vi "Do 6-Contact Sample Hall Calculations.vi"(8 "error in (no error)":errorcluster) -> (0 "error out":errorcluster)   [LabVIEW 2016, in "Hall Effect Library.lvlib"]
uses:
  Hall Effect Library.lvlib
  Global Variables/Hall Effect Data.vi
  Global Variables/Test Settings.vi
panel:
  out "uH":dbl
  out "Ravg":dbl
  out "Rh2":dbl
  out "Rh1":dbl
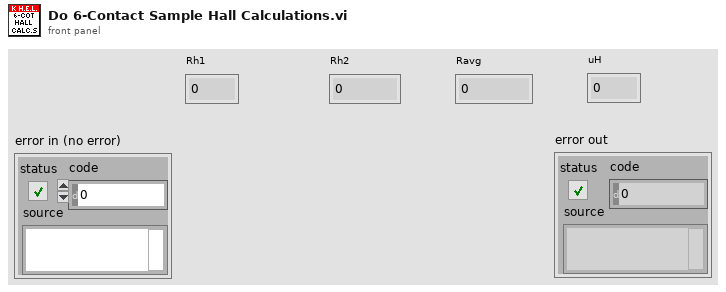
[diagram p1: front panel]
types:
  T1 = cluster{"RAvg":dbl, "RH1":dbl, "RH2":dbl, "uH":dbl}
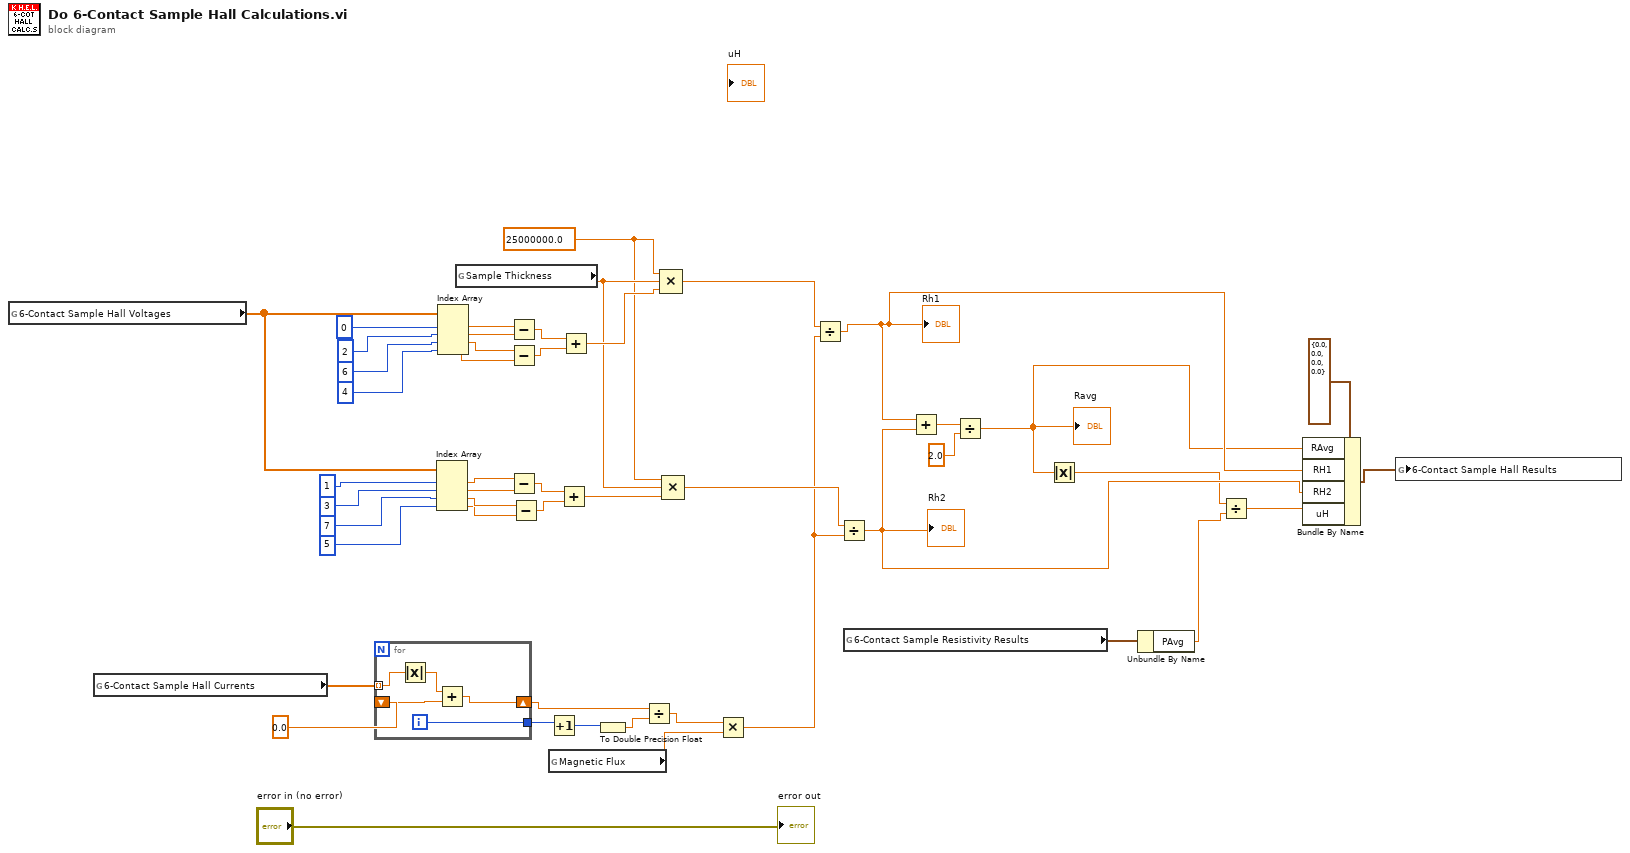
[diagram p0: block diagram]
diagram:
  w17 = 25000000.0
  n1 = global read "Hall Effect Data.vi" "6-Contact Sample Hall Voltages"() -> (w30:dbl[])
  n2 = global read "Hall Effect Data.vi" "6-Contact Sample Hall Currents"() -> (w46:dbl[])
  n3 = for {
    shift-right: [w52] -> w42
    shift-left: 0.0 -> [w53]
    tunnel: w46 -> [w50] mode=indexing
    tunnel: [w51] -> w45
    i -> [w51]
    n4 = Absolute Value(x=w50) -> (abs(x)=w49:dbl)
    n5 = Add(x=w49, y=w53) -> (x+y=w52:dbl)
  }
  n6 = Index Array(array=w30, index #1=1, index #2=3, index #3=7, index #4=5) -> (element #1=w25:dbl, element #2=w24:dbl, element #3=w23:dbl, element #4=w22:dbl)
  n7 = Index Array(array=w30, index #1=0, index #2=2, index #3=6, index #4=4) -> (element #1=w37:dbl, element #2=w36:dbl, element #3=w35:dbl, element #4=w34:dbl)
  n8 = global read "Test Settings.vi" "Sample Thickness"() -> (w18:dbl)
  n9 = Subtract(x=w37, y=w36) -> (x-y=w33:dbl)
  n10 = Subtract(x=w35, y=w34) -> (x-y=w32:dbl)
  n11 = Subtract(x=w25, y=w24) -> (x-y=w21:dbl)
  n12 = Subtract(x=w23, y=w22) -> (x-y=w20:dbl)
  n13 = Increment(x=w45) -> (x+1=w44:i32)
  n14 = global read "Test Settings.vi" "Magnetic Flux"() -> (w15:dbl)
  n15 = Add(x=w21, y=w20) -> (x+y=w19:dbl)
  n16 = Add(x=w33, y=w32) -> (x+y=w31:dbl)
  n17 = To Double Precision Float(number=w44) -> (double precision float=w43:dbl)
  n18 = Divide(x=w42, y=w43) -> (x/y=w16:dbl)
  n19 = Compound Arithmetic op=MULTIPLY(w17, w18, w31) -> (w14:dbl)
  n20 = Compound Arithmetic op=MULTIPLY(w17, w18, w19) -> (w13:dbl)
  n21 = Multiply(x=w16, y=w15) -> (x*y=w12:dbl)
  n22 = Divide(x=w14, y=w12) -> (x/y=w4:dbl)
  "Rh1" <- w4
  n23 = Divide(x=w13, y=w12) -> (x/y=w3:dbl)
  "Rh2" <- w3
  n24 = global read "Hall Effect Data.vi" "6-Contact Sample Resistivity Results"() -> (w9:cluster{"PAvg":dbl, "PA":dbl, "PB":dbl})
  n25 = Add(x=w4, y=w3) -> (x+y=w11:dbl)
  n26 = Divide(x=w11, y=2.0) -> (x/y=w2:dbl)
  "Ravg" <- w2
  n27 = Absolute Value(x=w2) -> (abs(x)=w1:dbl)
  n28 = Unbundle By Name(w9) -> ("PAvg"=w7:dbl)
  n29 = Divide(x=w1, y=w7) -> (x/y=w6:dbl)
  n30 = Bundle By Name(cluster=T1 {"RAvg"=0.0, "RH1"=0.0, "RH2"=0.0, "uH"=0.0} ("6-Contact Sample Hall Results"), "RAvg"=w2, "RH1"=w4, "RH2"=w3, "uH"=w6) -> (w5:T1)
  n31 = global write "Hall Effect Data.vi" "6-Contact Sample Hall Results"(w5) -> ()
  "error out" <- "error in (no error)"
